vi "rmad lyskontoll initfile.vi"(0 "init file":string="\\rmad config.ini", 11 "error in (no error)":errorcluster) -> (1 "num geophone nodes":u32, 2 "aktive skredløp":string[](array[string]), 3 "mast mot trafikklys output array":i32[](array[numeric]), 9 "sms enabled":bool, 10 "lights enables":bool, 12 "status":string[](array[string]), 13 "sms":string[](array[string]), 14 "Trafikkontroll terskelverdier":T1(array[cluster]), 15 "error out":errorcluster)   [LabVIEW 2017]
uses:
  <vilib>/Utility/config.llb/Read Key (Boolean).vi
  <vilib>/Utility/config.llb/Read Key (U32).vi
  <vilib>/Utility/config.llb/Read Key (I32).vi
  <vilib>/Utility/config.llb/NI_LVConfig.lvlib
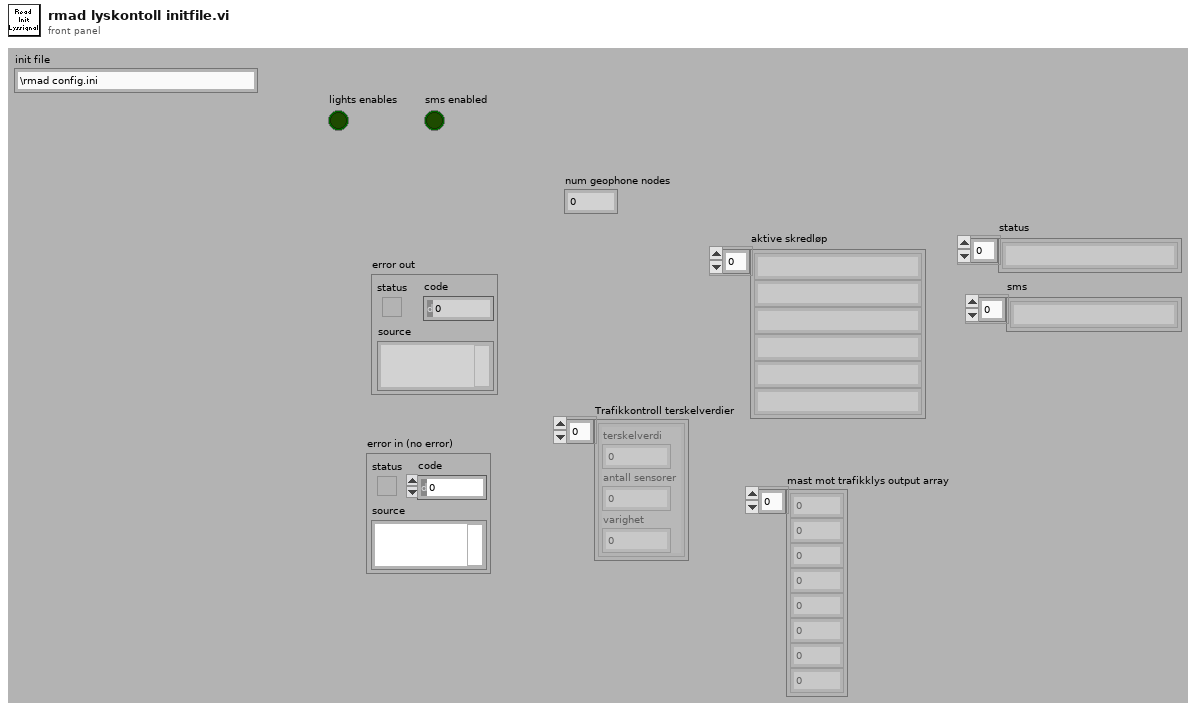
[diagram p1: front panel]
types:
  T1 = cluster{"terskelverdi":u32, "antall sensorer":u32, "varighet":u32}[]
  T2 = typedef "NI_LVConfig.lvlib/Config Data RefNum.ctl" = refnum<k1>
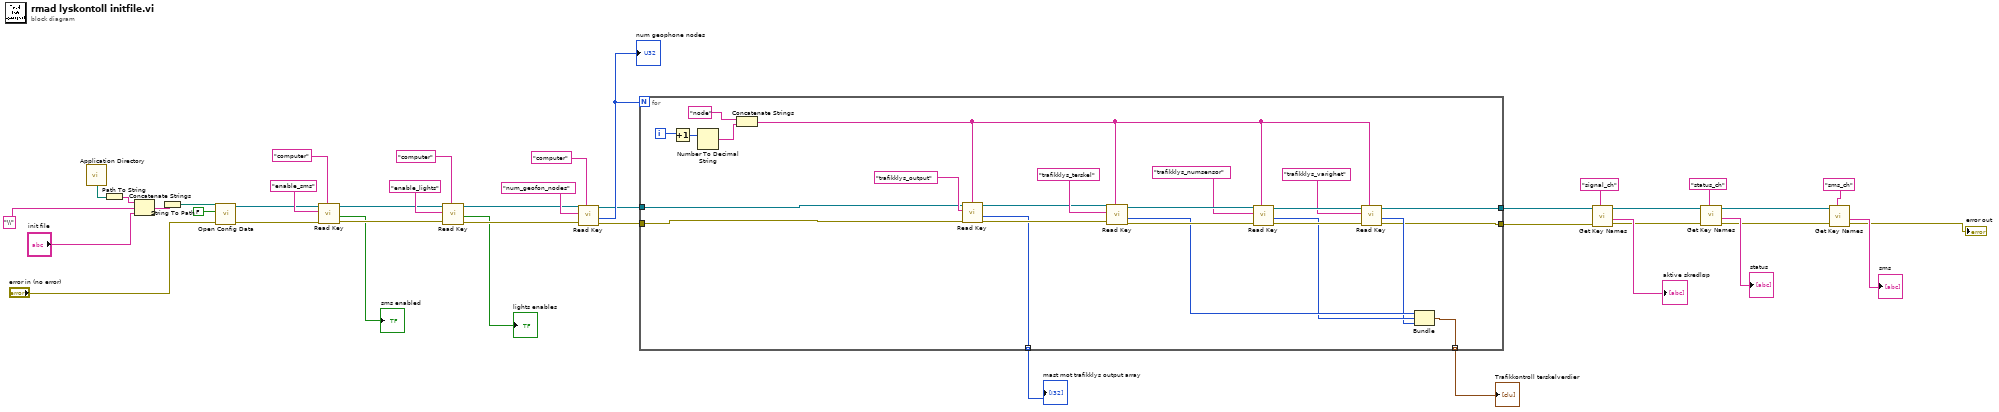
[diagram p0: block diagram]
diagram:
  n1 = call <vilib>:"Application Directory.vi"() -> ("Application Directory"=w40:path)
  n2 = Path To String(path=w40) -> (string=w39:string)
  n3 = Concatenate Strings(w39, "\\", "init file") -> (w37:string)
  n4 = String To Path(string=w37) -> (path=w36:path)
  n5 = call <vilib>:"Open Config Data.vi"("error in (no error)"="error in (no error)", "create file if necessary (T)"=FALSE, "configuration file path"=w36) -> ("error out"=w10:errorcluster, "refnum"=w11:T2)  [unwired: 6 in, 1 out]
  n6 = call-poly <vilib>:"Read Key.vi"("section"="computer", "error in (no error)"=w10, "key"="enable_sms", "refnum"=w11) -> ("error out"=w9:errorcluster, "value"=→"sms enabled":bool, "refnum out"=w8:T2)  [unwired: 4 in, 1 out]
  n7 = call-poly <vilib>:"Read Key.vi"("section"="computer", "error in (no error)"=w9, "key"="enable_lights", "refnum"=w8) -> ("error out"=w23:errorcluster, "value"=→"lights enables":bool, "refnum out"=w22:T2)  [unwired: 4 in, 1 out]
  n8 = call-poly <vilib>:"Read Key.vi"("section"="computer", "error in (no error)"=w23, "key"="num_geofon_nodes", "refnum"=w22) -> ("error out"=w31:errorcluster, "value"=w32:u32, "refnum out"=w30:T2)  [unwired: 4 in, 1 out]
  "num geophone nodes" <- w32
  n9 = for {
    N: w32 -> [_]
    tunnel: w31 -> [w41]
    tunnel: w30 -> [w42]
    tunnel: [w48] -> w28
    tunnel: [w49] -> w4
    tunnel: [w50] -> w3 mode=indexing
    tunnel: [w43] -> w1 mode=indexing
    i -> [w62]
    n10 = Increment(x=w62) -> (x+1=w61:i32)
    n11 = Number To Decimal String(number=w61) -> (decimal integer string=w63:string)  [unwired: 1 in]
    n12 = Concatenate Strings("node" ("string"), w63) -> (w45:string)
    n13 = call-poly <vilib>:"Read Key.vi"("section"=w45, "error in (no error)"=w41, "key"="trafikklys_output" ("section"), "refnum"=w42) -> ("error out"=w47:errorcluster, "value"=w43:i32, "refnum out"=w46:T2)  [unwired: 4 in, 1 out]
    n14 = call-poly <vilib>:"Read Key.vi"("section"=w45, "error in (no error)"=w47, "key"="trafikklys_terskel" ("section"), "refnum"=w46) -> ("error out"=w59:errorcluster, "value"=w53:u32, "refnum out"=w58:T2)  [unwired: 4 in, 1 out]
    n15 = call-poly <vilib>:"Read Key.vi"("section"=w45, "error in (no error)"=w59, "key"="trafikklys_numsensor", "refnum"=w58) -> ("error out"=w57:errorcluster, "value"=w52:u32, "refnum out"=w56:T2)  [unwired: 4 in, 1 out]
    n16 = call-poly <vilib>:"Read Key.vi"("section"=w45, "error in (no error)"=w57, "key"="trafikklys_varighet", "refnum"=w56) -> ("error out"=w49:errorcluster, "value"=w51:u32, "refnum out"=w48:T2)  [unwired: 4 in, 1 out]
    n17 = Bundle("value"=w53, "value"=w52, "value"=w51) -> (w50:cluster{"value":u32, "value":u32, "value":u32})  [unwired: 1 in]
  }
  "Trafikkontroll terskelverdier" <- w3
  "mast mot trafikklys output array" <- w1
  n18 = call <vilib>:"Get Key Names.vi"("section"="signal_ch", "error in (no error)"=w4, "refnum"=w28) -> ("error out"=w17:errorcluster, "key names"=→"aktive skredløp":string[], "refnum out"=w18:T2)  [unwired: 5 in, 1 out]
  n19 = call <vilib>:"Get Key Names.vi"("section"="status_ch", "error in (no error)"=w17, "refnum"=w18) -> ("error out"=w5:errorcluster, "key names"=→"status":string[], "refnum out"=w6:T2)  [unwired: 5 in, 1 out]
  n20 = call <vilib>:"Get Key Names.vi"("section"="sms_ch", "error in (no error)"=w5, "refnum"=w6) -> ("error out"=→"error out":errorcluster, "key names"=→"sms":string[])  [unwired: 5 in, 2 out]
